vi "sub_SDR_demod.vi"(10 "Input Symbols":cdb[](array[numeric]), 11 "Modulation Type":enum16{"BPSK", "4-QAM", "16-QAM", "64-QAM"}(ring)) -> (2 "Output bits":bool[](array[boolean]), 3 "SNR [dB]":dbl)   [LabVIEW 2012]
uses:
  <vilib>/Analysis/NI_AALBase.lvlib
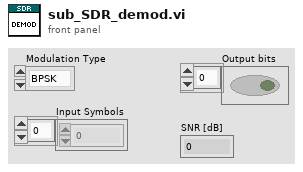
[diagram p1: front panel]
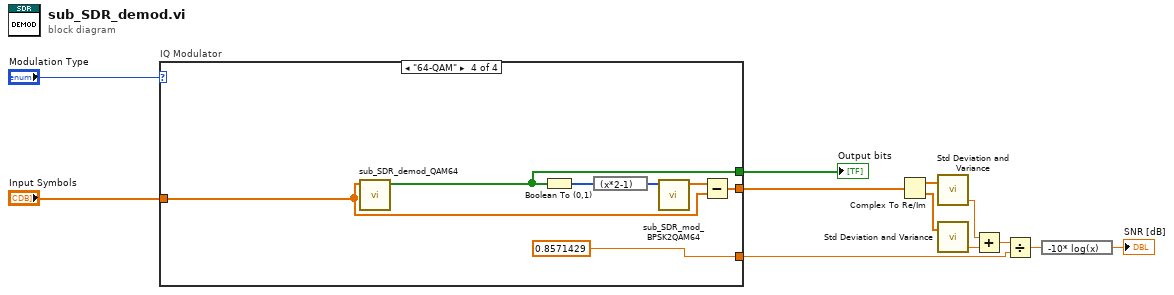
[diagram p0: block diagram]
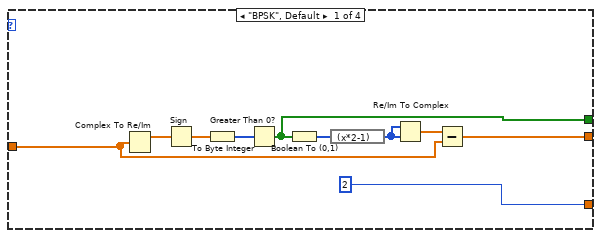
[diagram p2: hidden frame]
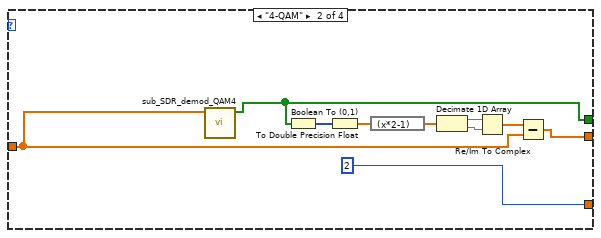
[diagram p3: hidden frame]
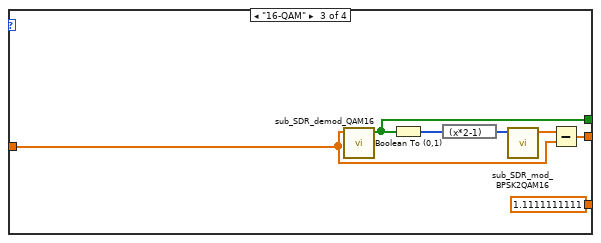
[diagram p4: hidden frame]
diagram:
  n1 = case "IQ Modulator" shown="\"64-QAM\"" "Modulation Type" {
    tunnel: "Input Symbols" -> [w17 w25 w35 w41]
    tunnel: [w15 w32 w39 w40] -> w1
    tunnel: [w14 w24 w36 w43] -> w7
    tunnel: [2 2 1.1111111111 0.8571429] -> w5
    frame "BPSK", Default {
      # "BPSK Modulator: Convert each input byte array into bolean arrays, sets phase and convert into complex"
      n2 = Complex To Re/Im(x + iy=w17) -> (x=w22:dbl[])  [unwired: 1 out]
      n3 = Sign(1:w22) -> (0:w21:dbl[])
      n4 = To Byte Integer(number=w21) -> (8bit integer=w20:i8[])
      n5 = Greater Than 0?(x=w20) -> (x > 0?=w15:bool[])
      n6 = Boolean To (0,1)(Boolean=w15) -> (0, 1=w13:i16[])
      n7 = expression code="(x*2-1)"(w13) -> (w16:i16[])
      n8 = Re/Im To Complex(1:w16, 2:w16) -> (0:w18:cdb[])
      n9 = Subtract(x=w18, y=w17) -> (x-y=w14:cdb[])
    }
    frame "4-QAM" {
      # "4-QAM Modulator: Convert each byte in 4 integers which are maped in the defined symbols"
      n10 = call "sub_SDR_demod_QAM4.vi"("Input Symbols"=w25) -> ("Demodulated data"=w32:bool[])  [unwired: 10 in]
      n11 = Boolean To (0,1)(Boolean=w32) -> (0, 1=w31:i16[])
      n12 = To Double Precision Float(number=w31) -> (double precision float=w30:dbl[])
      n13 = expression code="(x*2-1)"(w30) -> (w29:dbl[])
      n14 = Decimate 1D Array(w29) -> (w28:dbl[], w27:dbl[])
      n15 = Re/Im To Complex(1:w27, 2:w28) -> (0:w26:cdb[])
      n16 = Subtract(x=w26, y=w25) -> (x-y=w24:cdb[])
    }
    frame "16-QAM" {
      # "16-QAM Modulator: Convert each byte in 4 integers which are maped in a 4-MSK and build the phase and quadrature after"
      n17 = call "sub_SDR_demod_QAM16.vi"("Input Symbols"=w35) -> ("Array"=w39:bool[])  [unwired: 10 in]
      n18 = Boolean To (0,1)(Boolean=w39) -> (0, 1=w38:i16[])
      n19 = expression code="(x*2-1)"(w38) -> (w37:i16[])
      n20 = call "sub_SDR_mod_BPSK2QAM16.vi"("Array in"=w37) -> ("Array out"=w34:cdb[])  [unwired: 10 in]
      n21 = Subtract(x=w34, y=w35) -> (x-y=w36:cdb[])
    }
    frame "64-QAM" {
      n22 = call "sub_SDR_demod_QAM64.vi"("Input Symbols"=w41) -> ("Demodulated data"=w40:bool[])  [unwired: 10 in]
      n23 = Boolean To (0,1)(Boolean=w40) -> (0, 1=w46:i16[])
      n24 = expression code="(x*2-1)"(w46) -> (w45:i16[])
      n25 = call "sub_SDR_mod_BPSK2QAM64.vi"("Array in"=w45) -> ("Array out"=w44:cdb[])  [unwired: 10 in]
      n26 = Subtract(x=w44, y=w41) -> (x-y=w43:cdb[])
    }
  }
  "Output bits" <- w1
  n27 = Complex To Re/Im(x + iy=w7) -> (x=w8:dbl[], y=w9:dbl[])
  n28 = call <vilib>:"Std Deviation and Variance.vi"("X"=w8) -> ("variance"=w10:dbl)  [unwired: 1 in, 2 out]
  n29 = call <vilib>:"Std Deviation and Variance.vi"("X"=w9) -> ("variance"=w11:dbl)  [unwired: 1 in, 2 out]
  n30 = Add(x=w10, y=w11) -> (x+y=w12:dbl)
  n31 = Divide(x=w12, y=w5) -> (x/y=w4:dbl)
  n32 = expression code="-10* log(x)"(w4) -> (→"SNR [dB]":dbl)
